vi "DAC_lock_in_send_commands.vi"(1 "Inst info":T1, 2 "Points":cluster{string, "data":u64, "data":dbl}, 3 "FPGA VI Reference In":T2) -> ()   [LabVIEW 2013]
uses:
  fpga-bitfile-ref.ctl
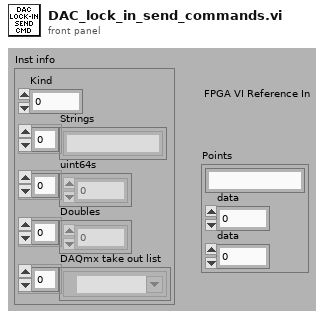
[diagram p1: front panel]
types:
  T1 = cluster{"Kind":u16, "Strings":string[], "uint64s":u64[], "Doubles":dbl[], "DAQmx take out list":refnum<k21>[]}
  T2 = typedef "fpga-bitfile-ref.ctl" = refnum<k20>
  T3 = enum16{"frequency", "channel", "amplitude", "inhibate"}
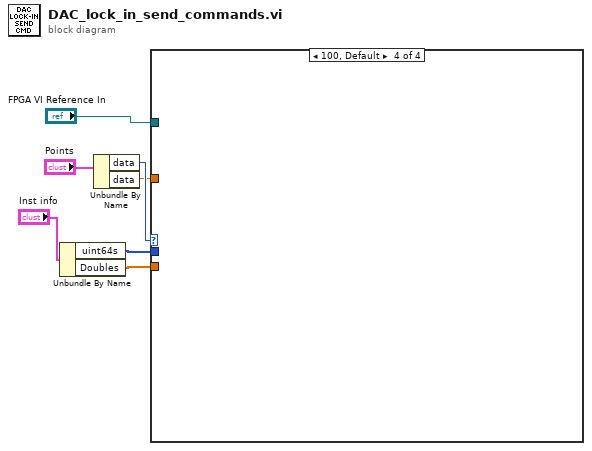
[diagram p0: block diagram]
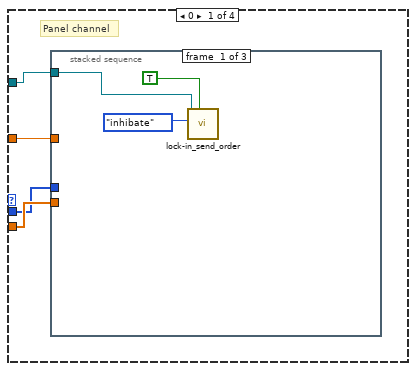
[diagram p2: hidden frame]
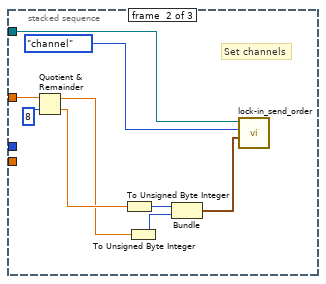
[diagram p3: hidden frame]
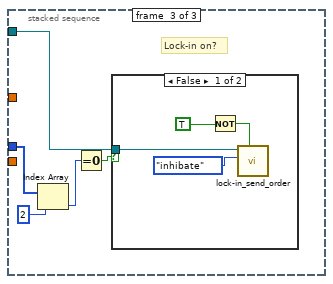
[diagram p4: hidden frame]
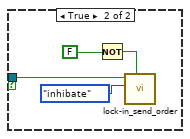
[diagram p5: hidden frame]
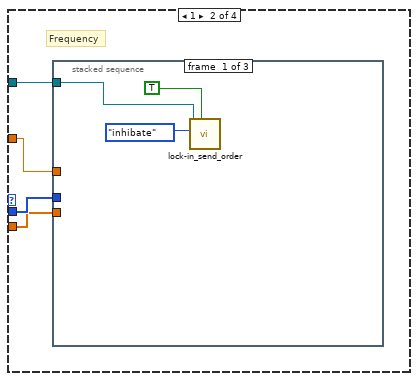
[diagram p6: hidden frame]
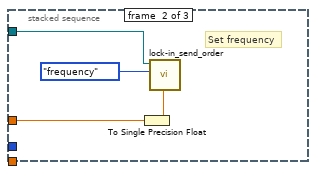
[diagram p7: hidden frame]
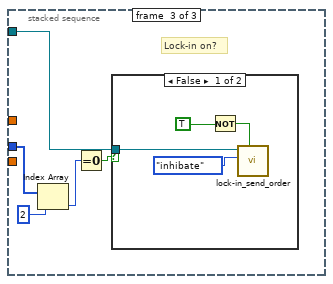
[diagram p8: hidden frame]
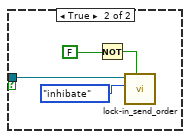
[diagram p9: hidden frame]
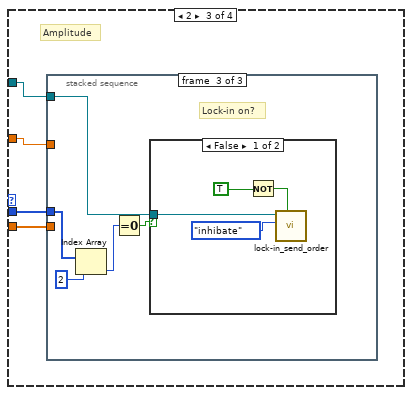
[diagram p10: hidden frame]
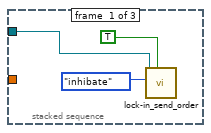
[diagram p11: hidden frame]
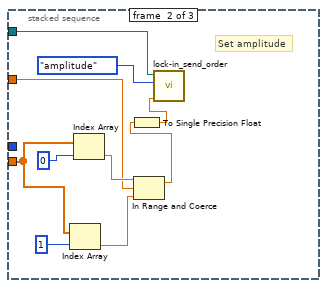
[diagram p12: hidden frame]
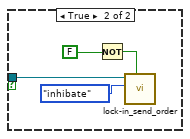
[diagram p13: hidden frame]
diagram:
  n1 = Unbundle By Name("Inst info") -> ("uint64s"=w5:u64[], "Doubles"=w4:dbl[])
  n2 = Unbundle By Name("Points") -> ("data"=w2:u64, "data"=w1:dbl)
  n3 = case shown="100, Default" w2 {
    tunnel: "FPGA VI Reference In" -> [w11 w40 w64 _]
    tunnel: w5 -> [w9 w39 w63 _]
    tunnel: w4 -> [w10 w38 w62 _]
    tunnel: w1 -> [w8 w37 w61 _]
    frame 0 {
      # "Panel channel"
      n4 = stacked-sequence {
        tunnel: w11 -> [w14 w23 w28]
        tunnel: w9 -> [_ _ w27]
        tunnel: w10 -> [_ _ _]
        tunnel: w8 -> [_ w18 _]
        frame #0 {
          n5 = call "lock-in_send_order.vi"("inhibate?"=TRUE, "order"=T3."inhibate", "FPGA VI Reference In"=w14) -> ()  [unwired: 4 in, 5 out]
        }
        frame #1 {
          # "Set channels"
          n6 = Quotient & Remainder(x=w18, y=8) -> (x-y*floor(x/y)=w15:dbl, floor(x/y)=w16:dbl)
          n7 = To Unsigned Byte Integer(number=w16) -> (unsigned 8bit integer=w20:u8)
          n8 = To Unsigned Byte Integer(number=w15) -> (unsigned 8bit integer=w19:u8)
          n9 = Bundle(w20, w19) -> (w21:cluster{u8, u8})  [unwired: 1 in]
          n10 = call "lock-in_send_order.vi"("Chanel (cl)"=w21, "order"=T3."channel", "FPGA VI Reference In"=w23) -> ()  [unwired: 3 in, 6 out]
        }
        frame #2 {
          # "Lock-in on?"
          n11 = Index Array(array=w27, index=2) -> (element=w24:u64)
          n12 = Equal To 0?(x=w24) -> (x = 0?=w25:bool)
          n13 = case shown="False" w25 {
            tunnel: w28 -> [w29 w35]
            frame False {
              n14 = Not(x=TRUE) -> (.not. x?=w31:bool)
              n15 = call "lock-in_send_order.vi"("inhibate?"=w31, "order"=T3."inhibate", "FPGA VI Reference In"=w29) -> ()  [unwired: 4 in, 5 out]
            }
            frame True {
              n16 = Not(x=FALSE) -> (.not. x?=w34:bool)
              n17 = call "lock-in_send_order.vi"("inhibate?"=w34, "order"=T3."inhibate", "FPGA VI Reference In"=w35) -> ()  [unwired: 4 in, 5 out]
            }
          }
        }
      }
    }
    frame 1 {
      # "Frequency"
      n18 = stacked-sequence {
        tunnel: w40 -> [w43 w46 w52]
        tunnel: w39 -> [_ _ w51]
        tunnel: w38 -> [_ _ _]
        tunnel: w37 -> [_ w44 _]
        frame #0 {
          n19 = call "lock-in_send_order.vi"("inhibate?"=TRUE, "order"=T3."inhibate", "FPGA VI Reference In"=w43) -> ()  [unwired: 4 in, 5 out]
        }
        frame #1 {
          # "Set frequency"
          n20 = To Single Precision Float(number=w44) -> (single precision float=w45:sgl)
          n21 = call "lock-in_send_order.vi"("frequency (Hz)"=w45, "order"=T3."frequency", "FPGA VI Reference In"=w46) -> ()  [unwired: 3 in, 6 out]
        }
        frame #2 {
          # "Lock-in on?"
          n22 = Index Array(array=w51, index=2) -> (element=w48:u64)
          n23 = Equal To 0?(x=w48) -> (x = 0?=w49:bool)
          n24 = case shown="False" w49 {
            tunnel: w52 -> [w53 w59]
            frame False {
              n25 = Not(x=TRUE) -> (.not. x?=w55:bool)
              n26 = call "lock-in_send_order.vi"("inhibate?"=w55, "order"=T3."inhibate", "FPGA VI Reference In"=w53) -> ()  [unwired: 4 in, 5 out]
            }
            frame True {
              n27 = Not(x=FALSE) -> (.not. x?=w58:bool)
              n28 = call "lock-in_send_order.vi"("inhibate?"=w58, "order"=T3."inhibate", "FPGA VI Reference In"=w59) -> ()  [unwired: 4 in, 5 out]
            }
          }
        }
      }
    }
    frame 2 {
      # "Amplitude"
      n29 = stacked-sequence {
        tunnel: w64 -> [w67 w76 w82]
        tunnel: w63 -> [_ _ w81]
        tunnel: w62 -> [_ w75 _]
        tunnel: w61 -> [_ w68 _]
        frame #0 {
          n30 = call "lock-in_send_order.vi"("inhibate?"=TRUE, "order"=T3."inhibate", "FPGA VI Reference In"=w67) -> ()  [unwired: 4 in, 5 out]
        }
        frame #1 {
          # "Set amplitude"
          n31 = Index Array(array=w75, index=1) -> (element=w73:dbl)
          n32 = Index Array(array=w75, index=0) -> (element=w74:dbl)
          n33 = In Range and Coerce(upper limit=w74, x=w68, lower limit=w73) -> (coerced(x)=w72:dbl)  [unwired: 1 out]
          n34 = To Single Precision Float(number=w72) -> (single precision float=w71:sgl)
          n35 = call "lock-in_send_order.vi"("amplitude"=w71, "order"=T3."amplitude", "FPGA VI Reference In"=w76) -> ()  [unwired: 3 in, 6 out]
        }
        frame #2 {
          # "Lock-in on?"
          n36 = Index Array(array=w81, index=2) -> (element=w78:u64)
          n37 = Equal To 0?(x=w78) -> (x = 0?=w79:bool)
          n38 = case shown="False" w79 {
            tunnel: w82 -> [w83 w89]
            frame False {
              n39 = Not(x=TRUE) -> (.not. x?=w85:bool)
              n40 = call "lock-in_send_order.vi"("inhibate?"=w85, "order"=T3."inhibate", "FPGA VI Reference In"=w83) -> ()  [unwired: 4 in, 5 out]
            }
            frame True {
              n41 = Not(x=FALSE) -> (.not. x?=w88:bool)
              n42 = call "lock-in_send_order.vi"("inhibate?"=w88, "order"=T3."inhibate", "FPGA VI Reference In"=w89) -> ()  [unwired: 4 in, 5 out]
            }
          }
        }
      }
    }
    frame 100, Default {
    }
  }
